vi "Manage battery alert.vi"(7 "Application path":path, 8 "Error In":errorcluster, 10 "Vbattery":dbl min=0.0 max=4.2 step=0.05 format="%#.2gV", 11 "MAC address":string) -> (0 "Error Out":errorcluster)   [LabVIEW 2016]
uses:
  <vilib>/Utility/config.llb/Read Key (Boolean).vi
  <vilib>/Utility/config.llb/Read Key (Double).vi
  <vilib>/Utility/config.llb/Read Key (String).vi
  <vilib>/Utility/config.llb/Write Key (Double).vi
  <vilib>/Utility/SMTP/NI_SMTPEmail.lvlib
  <vilib>/Utility/config.llb/NI_LVConfig.lvlib
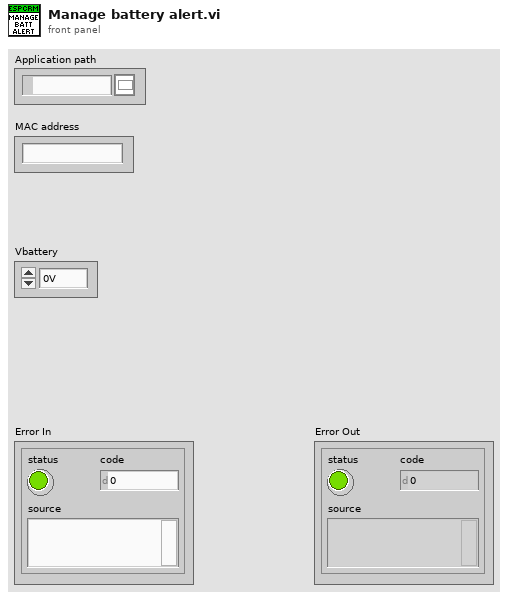
[diagram p1: front panel]
types:
  T1 = typedef "NI_LVConfig.lvlib/Config Data RefNum.ctl" = refnum<k1>
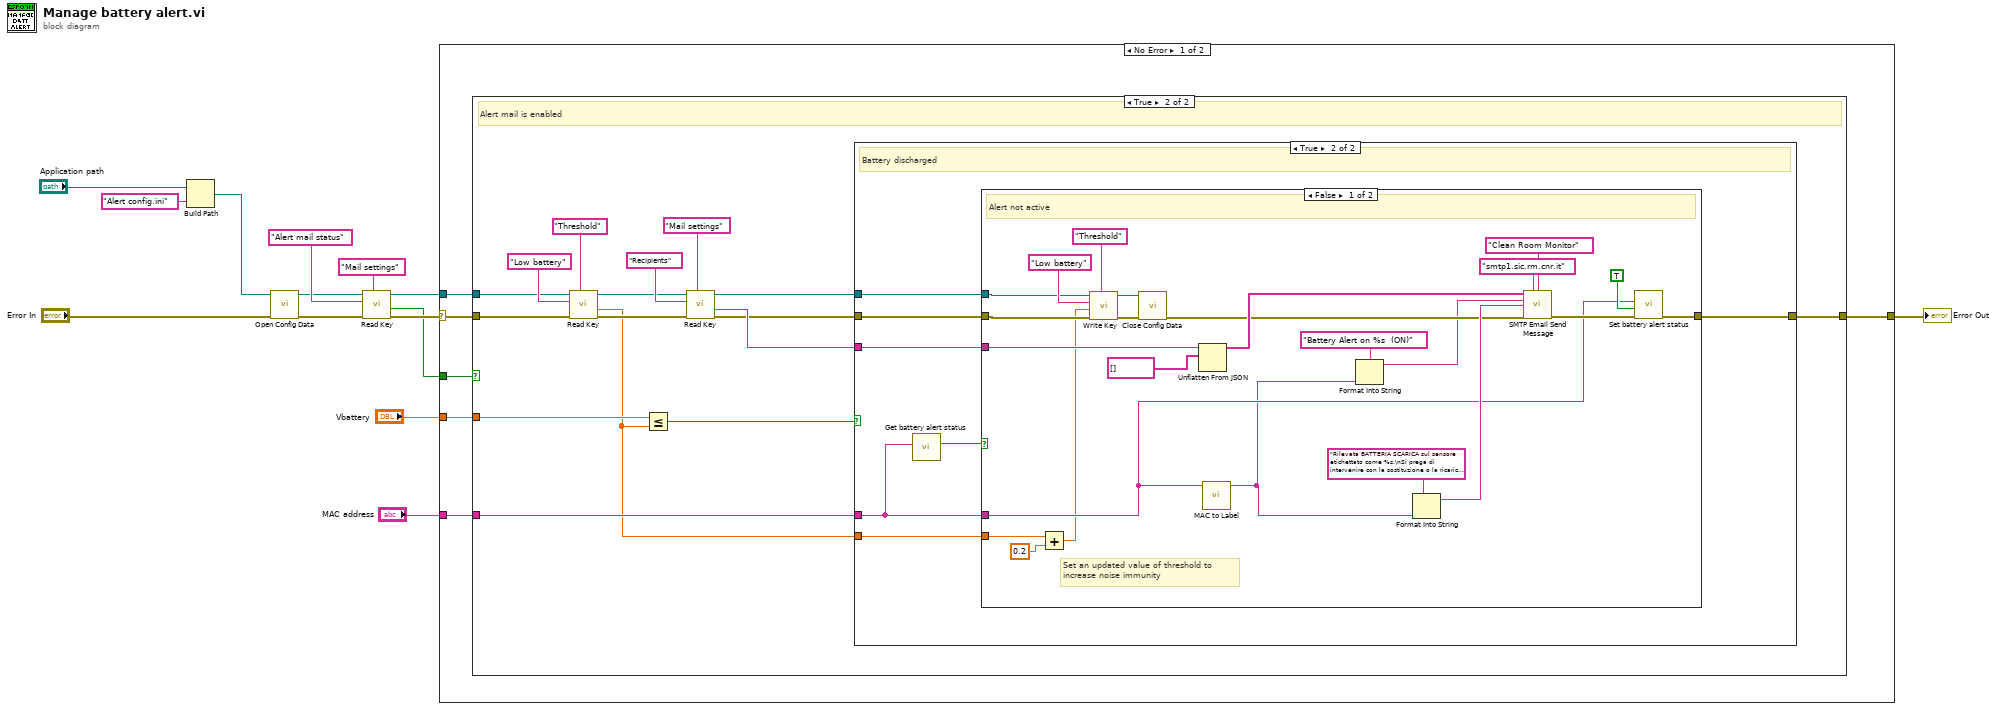
[diagram p0: block diagram]
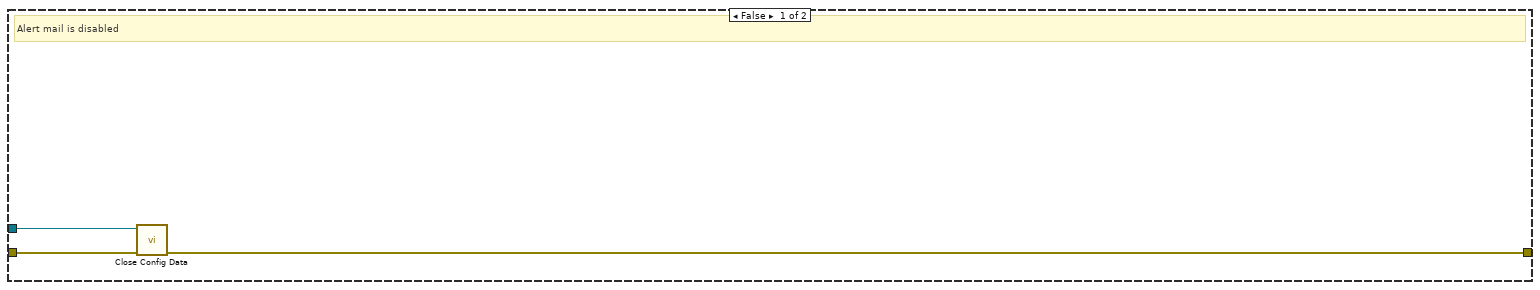
[diagram p2: hidden frame]
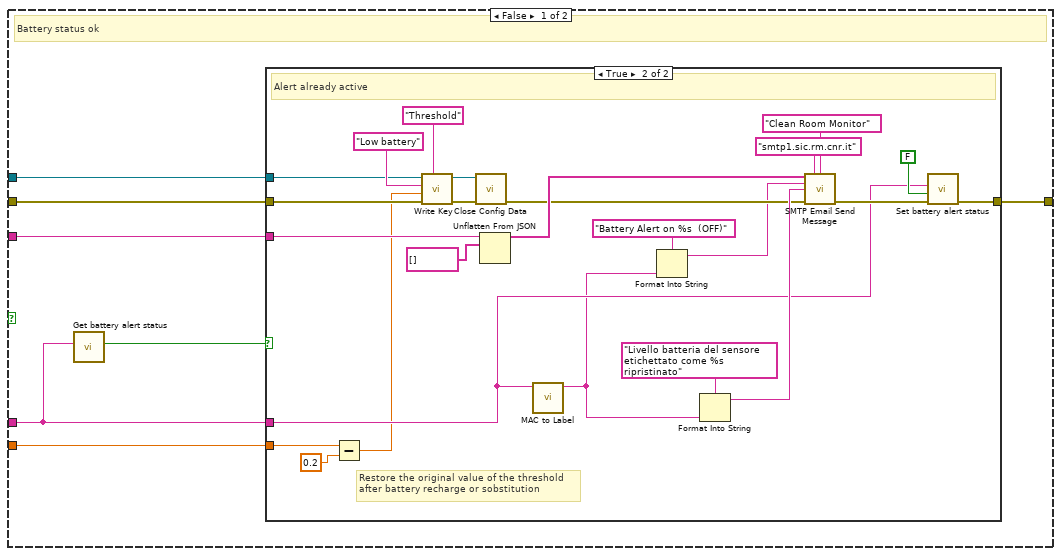
[diagram p3: hidden frame]
diagram:
  n1 = Build Path(base path="Application path", name or relative path="Alert config.ini") -> (appended path=w13:path)
  n2 = call <vilib>:"Open Config Data.vi"("error in (no error)"="Error In", "configuration file path"=w13) -> ("error out"=w8:errorcluster, "refnum"=w9:T1)  [unwired: 7 in, 1 out]
  n3 = call-poly <vilib>:"Read Key.vi"("section"="Mail settings", "error in (no error)"=w8, "key"="Alert mail status", "refnum"=w9) -> ("error out"=w6:errorcluster, "value"=w4:bool, "refnum out"=w7:T1)  [unwired: 4 in, 1 out]
  n4 = case shown="No Error" w6 {
    selector: w6 -> [w19 w104]
    tunnel: [w16 w104] -> w14
    tunnel: w7 -> [w18 _]
    tunnel: w4 -> [w20 _]
    tunnel: "Vbattery" -> [w17 _]
    tunnel: "MAC address" -> [w15 _]
    frame No Error {
      n5 = case shown="True" w20 {
        tunnel: w19 -> [w23 w34]
        tunnel: w18 -> [w21 w35]
        tunnel: w17 -> [_ w30]
        tunnel: [w22 w33] -> w16
        tunnel: w15 -> [_ w32]
        frame False {
          # "Alert mail is disabled"
          n6 = call <vilib>:"Close Config Data.vi"("error in (no error)"=w23, "refnum"=w21) -> ("error out"=w22:errorcluster)  [unwired: 8 in, 1 out]
        }
        frame True {
          # "Alert mail is enabled"
          n7 = call-poly <vilib>:"Read Key.vi"("section"="Threshold", "error in (no error)"=w34, "key"="Low battery", "refnum"=w35) -> ("error out"=w28:errorcluster, "value"=w26:dbl, "refnum out"=w29:T1)  [unwired: 4 in, 1 out]
          n8 = Less Or Equal?(x=w30, y=w26) -> (x <= y?=w27:bool)
          n9 = call-poly <vilib>:"Read Key.vi"("section"="Mail settings", "error in (no error)"=w28, "key"="Recipients", "refnum"=w29) -> ("error out"=w25:errorcluster, "value"=w31:string, "refnum out"=w24:T1)  [unwired: 4 in, 1 out]
          n10 = case shown="True" w27 {
            tunnel: w25 -> [w45 w78]
            tunnel: [w42 w77] -> w33
            tunnel: w32 -> [w43 w75]
            tunnel: w31 -> [w44 w76]
            tunnel: w26 -> [w41 w72]
            tunnel: w24 -> [w40 w73]
            frame False {
              # "Battery status ok"
              n11 = call "Get battery alert status.vi"("MAC address"=w43) -> ("Is Alert Active?"=w46:bool)  [unwired: 9 in, 1 out]
              n12 = case shown="True" w46 {
                tunnel: w45 -> [w47 w53]
                tunnel: [w47 w64] -> w42
                tunnel: w43 -> [_ w62]
                tunnel: w44 -> [_ w69]
                tunnel: w41 -> [_ w59]
                tunnel: w40 -> [_ w54]
                frame False {
                  # "Alert not active"
                }
                frame True {
                  # "Restore the original value of the threshold\nafter battery recharge or sobstitution"
                  # "Alert already active"
                  n13 = Subtract(x=w59, y=0.2) -> (x-y=w51:dbl)
                  n14 = call-poly <vilib>:"Write Key.vi"("section"="Threshold", "error in (no error)"=w53, "value"=w51, "key"="Low battery", "refnum"=w54) -> ("error out"=w56:errorcluster, "refnum out"=w55:T1)  [unwired: 4 in, 1 out]
                  n15 = call <vilib>:"Close Config Data.vi"("error in (no error)"=w56, "refnum"=w55) -> ("error out"=w52:errorcluster)  [unwired: 8 in, 1 out]
                  n16 = Unflatten From JSON(JSON string=w69, type and defaults=string[] []) -> (value=w67:string[])  [unwired: 5 in, 1 out]
                  n17 = call "MAC to Label.vi"("MAC address"=w62) -> ("Label"=w49:string)  [unwired: 9 in, 1 out]
                  n18 = Format Into String(format string="Battery Alert on %s  (OFF)" ("subject ([No Subject])"), w49) -> (resulting string=w48:string)  [unwired: 2 in, 1 out]
                  n19 = Format Into String(format string="Livello batteria del sensore etichettato come %s ripristinato", w49) -> (resulting string=w70:string)  [unwired: 2 in, 1 out]
                  n20 = call <vilib>:"SMTP Email Send Message.vi"("recipients"=w67, "mail server"="smtp1.sic.rm.cnr.it" ("Mail Server 2"), "return address"="Clean Room Monitor", "subject ([No Subject])"=w48, "message"=w70, "error in (no error)"=w52) -> ("error out"=w65:errorcluster)  [unwired: 8 in, 1 out]
                  n21 = call "Set battery alert status.vi"("Error In"=w65, "Alert status"=FALSE, "MAC address"=w62) -> ("Error Out"=w64:errorcluster)  [unwired: 7 in]
                }
              }
            }
            frame True {
              # "Battery discharged"
              n22 = call "Get battery alert status.vi"("MAC address"=w75) -> ("Is Alert Active?"=w74:bool)  [unwired: 9 in, 1 out]
              n23 = case shown="False" w74 {
                tunnel: w78 -> [w88 w103]
                tunnel: [w94 w103] -> w77
                tunnel: w75 -> [w92 _]
                tunnel: w76 -> [w99 _]
                tunnel: w73 -> [w89 _]
                tunnel: w72 -> [w86 _]
                frame False {
                  # "Set an updated value of threshold to \nincrease noise immunity"
                  # "Alert not active"
                  n24 = Add(x=w86, y=0.2) -> (x+y=w85:dbl)
                  n25 = call-poly <vilib>:"Write Key.vi"("section"="Threshold", "error in (no error)"=w88, "value"=w85, "key"="Low battery", "refnum"=w89) -> ("error out"=w84:errorcluster, "refnum out"=w83:T1)  [unwired: 4 in, 1 out]
                  n26 = call <vilib>:"Close Config Data.vi"("error in (no error)"=w84, "refnum"=w83) -> ("error out"=w82:errorcluster)  [unwired: 8 in, 1 out]
                  n27 = Unflatten From JSON(JSON string=w99, type and defaults=string[] []) -> (value=w97:string[])  [unwired: 5 in, 1 out]
                  n28 = call "MAC to Label.vi"("MAC address"=w92) -> ("Label"=w80:string)  [unwired: 9 in, 1 out]
                  n29 = Format Into String(format string="Battery Alert on %s  (ON)" ("subject ([No Subject])"), w80) -> (resulting string=w79:string)  [unwired: 2 in, 1 out]
                  n30 = Format Into String(format string="Rilevata BATTERIA SCARICA sul sensore etichettato come %s.\nSi prega di intervenire con la sostituzione o la ricarica della batteria.", w80) -> (resulting string=w100:string)  [unwired: 2 in, 1 out]
                  n31 = call <vilib>:"SMTP Email Send Message.vi"("recipients"=w97, "mail server"="smtp1.sic.rm.cnr.it" ("Mail Server 2"), "return address"="Clean Room Monitor", "subject ([No Subject])"=w79, "message"=w100, "error in (no error)"=w82) -> ("error out"=w95:errorcluster)  [unwired: 8 in, 1 out]
                  n32 = call "Set battery alert status.vi"("Error In"=w95, "Alert status"=TRUE, "MAC address"=w92) -> ("Error Out"=w94:errorcluster)  [unwired: 7 in]
                }
                frame True {
                  # "Alert already active"
                }
              }
            }
          }
        }
      }
    }
    frame Error {
    }
  }
  "Error Out" <- w14
